vi "gentec-SOLO_PE.Close Connection.vi"(4 "error in":errorcluster, 7 "VISA resource name in":refnum<visa-resource-name>) -> (0 "error out":errorcluster)   [LabVIEW 2014, in "gentec-SOLO-PE - Driver.lvlib"]
doc: "This VI closes a VISA connection."
uses:
  gentec-SOLO-PE - Driver.lvlib
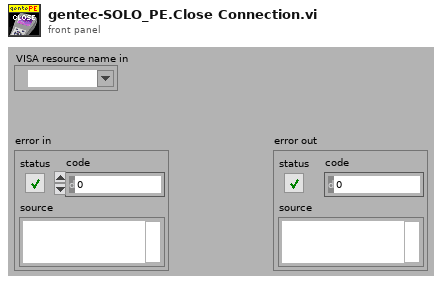
[diagram p1: front panel]
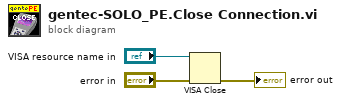
[diagram p0: block diagram]
diagram:
  n1 = VISA Close(VISA resource name="VISA resource name in", error in (no error)="error in") -> (error out=→"error out":errorcluster)
